vi "Show Hide (Label).vi"(5 "Invert? [F]":bool, 7 "Regex? [F]":bool, 8 "error in (no error)":errorcluster, 9 "Show? [T]":bool=TRUE, 10 "Label":string, 11 "MMI Scaling in":refnum<class "IObject.lvclass">) -> (0 "error out":errorcluster, 2 "Match?":bool, 3 "MMI Scaling out":refnum<class "IObject.lvclass">)   [LabVIEW 2021, in "IObject.lvclass"]
uses:
  IObject.lvclass
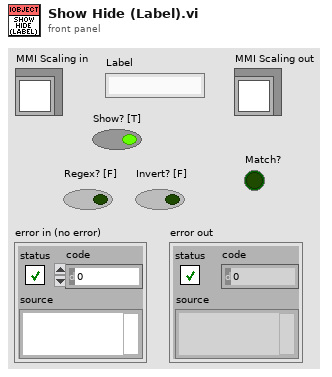
[diagram p1: front panel]
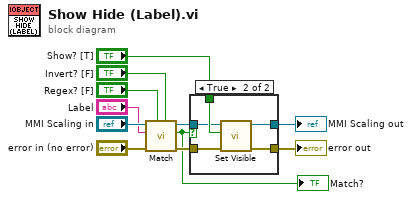
[diagram p0: block diagram]
diagram:
  n1 = call "Match.vi"("Invert? [F]"="Invert? [F]", "Regex? [F]"="Regex? [F]", "error in (no error)"="error in (no error)", "Label"="Label", "MMI Scaling in"="MMI Scaling in") -> ("error out"=w10:errorcluster, "Match?"=w1:bool, "MMI Scaling out"=w7:refnum<class "IObject.lvclass">)  [unwired: 4 in]
  "Match?" <- w1
  n2 = case shown="True" w1 {
    tunnel: w10 -> [w13 w17]
    tunnel: [w13 w15] -> w3
    tunnel: w7 -> [w12 w16]
    tunnel: [w12 w14] -> w2
    tunnel: "Show? [T]" -> [_ w18]
    frame False {
    }
    frame True {
      n3 = call-dynamic "Set Visible.vi"("error in (no error)"=w17, "Show? [T]"=w18, "MMI Scaling in"=w16) -> ("error out"=w15:errorcluster, "MMI Scaling out"=w14:refnum<class "IObject.lvclass">)  [unwired: 7 in]
    }
  }
  "error out" <- w3
  "MMI Scaling out" <- w2
